vi "刷新.vi"(8 "错误输入（无错误）":errorcluster, 11 "XY图输入":refnum<vi>) -> (0 "错误输出":errorcluster)   [LabVIEW 2021]
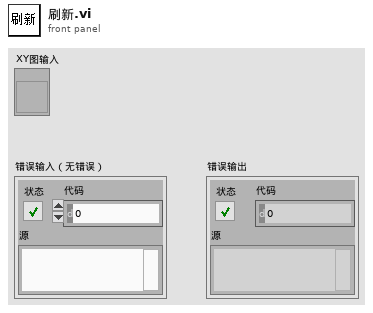
[diagram p1: front panel]
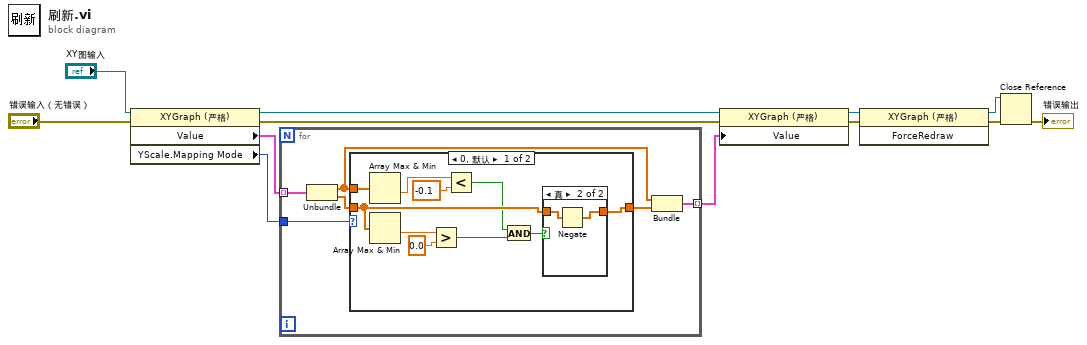
[diagram p0: block diagram]
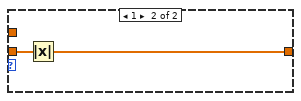
[diagram p3: hidden frame]
diagram:
  n1 = property class="XYGraph (严格)"(reference="XY图输入", error in="错误输入（无错误）") -> (reference out=w7:refnum<vi>, error out=w6:errorcluster, "Value"=w10:cluster{"测试数据":dbl[], "测试数据":dbl[]}[], "YScale.Mapping Mode"=w9:u8)
  n2 = for {
    tunnel: w10 -> [w18] mode=indexing
    tunnel: w9 -> [w17]
    tunnel: [w14] -> w8 mode=indexing
    n3 = Unbundle(w18) -> ("测试数据"=w13:dbl[], "测试数据"=w16:dbl[])
    n4 = case shown="0, 默认" w17 {
      tunnel: w16 -> [w24 w33]
      tunnel: [w23 w32] -> w15
      tunnel: w13 -> [w20 _]
      frame 0, Default {
        n5 = Array Max & Min(array=w20) -> (min value=w22:dbl)  [unwired: 3 out]
        n6 = Array Max & Min(array=w24) -> (min value=w27:dbl)  [unwired: 3 out]
        n7 = Greater?(x=w27, y=0.0) -> (0:w26:bool)
        n8 = Less?(x=w22, y=-0.1) -> (x < y?=w19:bool)
        n9 = And(x=w19, y=w26) -> (x .and. y?=w25:bool)
        n10 = case shown="真" w25 {
          tunnel: w24 -> [w29 w31]
          tunnel: [w29 w30] -> w23
          frame False {
          }
          frame True {
            n11 = Negate(x=w31) -> (-x=w30:dbl[])
          }
        }
      }
      frame 1 {
        n12 = Absolute Value(x=w33) -> (abs(x)=w32:dbl[])
      }
    }
    n13 = Bundle("测试数据"=w13, "测试数据"=w15) -> (w14:cluster{"测试数据":dbl[], "测试数据":dbl[]})  [unwired: 1 in]
  }
  n14 = property class="XYGraph (严格)"(reference=w7, error in=w6, "Value"=w8) -> (reference out=w5:refnum<vi>, error out=w4:errorcluster)
  n15 = invoke class="XYGraph (严格)" method="ForceRedraw"(reference=w5, error in=w4) -> (reference out=w1:refnum<vi>, error out=w3:errorcluster)  [unwired: 1 in, 1 out]
  n16 = Close Reference(reference=w1, error in (no error)=w3) -> (error out=→"错误输出":errorcluster)
